vi "4 - DAQmx Bus Digital Input and Output.vi"() -> ()   [LabVIEW 2021]
uses:
  <vilib>/TSA/Omni-Bus/Omni-Bus/Omni_Bus.lvclass
  <vilib>/TSA/Omni-Bus/Omni-Bus/Support/Broad Types.ctl
  <vilib>/TSA/Abstract Data Classes/Abs_Types/Type/Abs_Type.lvclass/Abs_Type.ctl
  <vilib>/TSA/Omni-Bus/Omni-Bus/Omni_Bus.lvclass/Omni_Bus.ctl
  <vilib>/TSA/Omni-Bus/Omni-Bus/Support/Read/Read Boolean.vi
  <vilib>/TSA/Omni-Bus/Omni-Bus/Support/Write/Write Boolean.vi
  <vilib>/TSA/Omni-Bus/Omni-Bus/Support/FindVar.vi
  <vilib>/Utility/error.llb/Clear Errors.vi
  <vilib>/TSA/Omni-Bus/Omni-Bus/Properties/Read Var Map.vi
  <vilib>/TSA/Abstract Data Classes/Abs_Types/Type/Properties/Read Tag.vi
  DAQmx-Bus.lvclass
  C:/Program Files (x86)/National Instruments/LabVIEW 2021/vi.lib/TSA/Omni-Bus/Omni-Bus/Bus Access/Bus_Access.lvclass
  <vilib>/TSA/Abstract Data Classes/Abs_Types/Boolean/Abs_Boolean.lvclass
  C:/Program Files (x86)/National Instruments/LabVIEW 2021/vi.lib/TSA/Abstract Data Classes/Abs_Types/Type/Abs_Type.lvclass
  <vilib>/TSA/Abstract Data Classes/Abs_Types/Value/Abs_Value.lvclass
  <vilib>/TSA/Omni-Bus/Omni-Bus/Support/Check For Read Only Error.vi
  <vilib>/TSA/Omni-Bus/Omni-Bus/Support/Incorrect Tag String Error.vi
  <vilib>/TSA/Abstract Data Classes/Abs_Types/Type/Abs_Type.lvclass
panel:
  in  "DAQmx In Task":refnum<k21>="Digital Input"
  in  "DAQmx Out Task":refnum<k21>="Digital Out"
  out "error out":errorcluster
  in  "Digital Out":bool
  in  "Digital Output Tag":string(combo)
  out "Digital In":bool
  out "timed out?":bool
  in  "stop":bool
  in  "Digital Input Tag":string(combo)
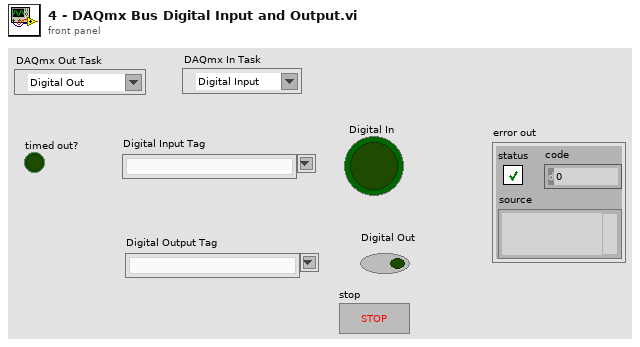
[diagram p1: front panel]
types:
  T1 = typedef "Omni_Bus.lvclass/Broad Types.ctl" = enum16{"All Tags", "NI Specific Type", "Boolean", "String", "Numeric", "Float", "Integer", "Collection", "All Value Types", "Non Value Types"}
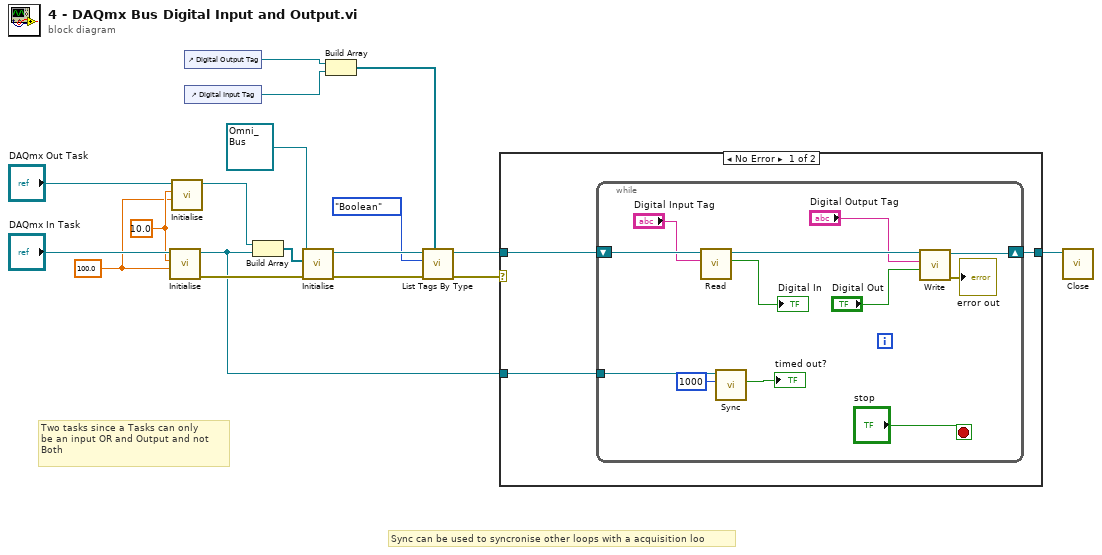
[diagram p0: block diagram]
diagram:
  w1 = 100.0 ("Update Rate (Hz) - Non HW Timed")
  w2 = 10.0 ("timeout")
  # "Sync can be used to syncronise other loops with a acquisition loo"
  # "Two tasks since a Tasks can only\nbe an input OR and Output and not\nBoth"
  n1 = call "Initialise.vi"("Update Rate (Hz) - Non HW Timed"=w1, "timeout (s)"=w2, "DAQmx Task"="DAQmx In Task") -> ("error out"=w16:errorcluster, "DAQmx-Bus out"=w9:refnum<class "DAQmx-Bus.lvclass">)  [unwired: 7 in]
  n2 = call "Initialise.vi"("Update Rate (Hz) - Non HW Timed"=w1, "timeout (s)"=w2, "DAQmx Task"="DAQmx Out Task") -> ("DAQmx-Bus out"=w7:refnum<class "DAQmx-Bus.lvclass">)  [unwired: 7 in, 1 out]
  n3 = control-ref of="Digital Output Tag"() -> (w6:refnum<vi>)
  n4 = control-ref of="Digital Input Tag"() -> (w5:refnum<vi>)
  n5 = Build Array(w7, w9) -> (w18:refnum<class "DAQmx-Bus.lvclass">[])
  n6 = call-dynamic "Initialise.vi"("error in (no error)"=w16, "Bus Access"=w18, "Var Bus in"=refnum<class "Omni_Bus.lvclass"> refnum) -> ("error out"=w13:errorcluster, "Var Bus out"=w14:refnum<class "Omni_Bus.lvclass">)  [unwired: 7 in]
  n7 = Build Array(w6, w5) -> (w4:refnum<vi>[])
  n8 = call <vilib>:"List Tags By Type.vi"("Combo Boxes"=w4, "error in (no error)"=w13, "Broad Types"=Broad_Types."Boolean", "Var Bus in"=w14) -> ("error out"=w11:errorcluster, "Var Bus out"=w12:refnum<class "Omni_Bus.lvclass">)  [unwired: 4 in, 2 out]
  n9 = case shown="No Error" w11 {
    tunnel: [w21 w34] -> w15
    tunnel: w12 -> [w20 w34]
    tunnel: w9 -> [w19 _]
    frame No Error {
      n10 = while {
        shift-right: [w25] -> w21
        shift-left: w20 -> [w33]
        tunnel: w19 -> [w30]
        stop <- "stop" stop-if-true
        n11 = call-poly <vilib>:"Read.vi"("Tag"="Digital Input Tag", "Var Bus in"=w33) -> ("Boolean"=→"Digital In":bool, "Var Bus out"=w26:refnum<class "Omni_Bus.lvclass">)  [unwired: 7 in, 1 out]
        n12 = call-dynamic "Sync.vi"("timeout in ms (-1)"=1000, "DAQmx-Bus in"=w30) -> ("timed out?"=→"timed out?":bool)  [unwired: 7 in, 2 out]
        n13 = call-poly <vilib>:"Write.vi"("Boolean"="Digital Out", "Tag"="Digital Output Tag", "Omni_Bus in"=w26) -> ("error out"=→"error out":errorcluster, "Omni_Bus out"=w25:refnum<class "Omni_Bus.lvclass">)  [unwired: 7 in]
      }
    }
    frame Error {
    }
  }
  n14 = call-dynamic "Close.vi"("Data in"=w15) -> ()  [unwired: 9 in, 2 out]
